vi "FT_Get_Com_Port_Number.vi"(0 "Handle":u32) -> (1 "FT_Status":u32, 2 "ComNumber":u32)   [LabVIEW 2019]
uses:
  FTD2XX.dll
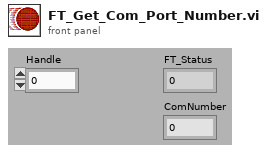
[diagram p1: front panel]
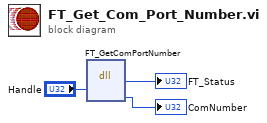
[diagram p0: block diagram]
diagram:
  n1 = dll-call lib="ftd2xx.dll" fn="FT_GetComPortNumber"("Handle"="Handle") -> ("FT_Status"=→"FT_Status":u32, "ComNumber"=→"ComNumber":i32)  [unwired: 5 in, 2 out]
